vi "MGI Dispose Daemon.vi"(11 "MGI Error Reporter Base In":refnum<class "MGI Error Reporter Base.lvclass">) -> (3 "MGI Error Reporter Base Out":refnum<class "MGI Error Reporter Base.lvclass">)   [LabVIEW 2020, in "MGI Error Reporter Base.lvclass"]
doc: "Releases the specified references. Child classes can perform other tasks as appropriate, but should use Call Parent Method before completing.\n\nAuthored by Shawn Walpole\nsupport@mooregoodideas.com\nwww.mooregoodideas.com\n\nCopyright (c) 2013, Moore Good Ideas, Inc.\n\nAll rights reserved.\n\nRedistribution and use in source and binary forms, with or without modification, are permitted provided that the following conditions are met:\n\n * Redistributions of source code must retain the above copyright notice, this list of conditions and the following disclaimer.\n * Redistributions in binary form must reproduce the above copyright notice, this list of conditions and the following disclaimer in the documentation and/or other materials provided with the distribution.\n * Neither the name of Moore Good Ideas, Inc. nor the names of its contributors may be used to endorse or promote products derived from this software without specific prior written permission.\n\nTHIS SOFTWARE IS PROVIDED BY THE COPYRIGHT HOLDERS AND CONTRIBUTORS \"AS IS\" AND ANY EXPRESS OR IMPLIED WARRANTIES, INCLUDING, BUT NOT LIMITED TO, THE IMPLIED WARRANTIES OF MERCHANTABILITY AND FITNESS FOR A PARTICULAR PURPOSE ARE DISCLAIMED. IN NO EVENT SHALL THE COPYRIGHT OWNER OR CONTRIBUTORS BE LIABLE FOR ANY DIRECT, INDIRECT, INCIDENTAL, SPECIAL, EXEMPLARY, OR CONSEQUENTIAL DAMAGES (INCLUDING, BUT NOT LIMITED TO, PROCUREMENT OF SUBSTITUTE GOODS OR SERVICES; LOSS OF USE, DATA, OR PROFITS; OR BUSINESS INTERRUPTION) HOWEVER CAUSED AND ON ANY THEORY OF LIABILITY, WHETHER IN CONTRACT, STRICT LIABILITY, OR TORT (INCLUDING NEGLIGENCE OR OTHERWISE) ARISING IN ANY WAY OUT OF THE USE OF THIS SOFTWARE, EVEN IF ADVISED OF THE POSSIBILITY OF SUCH DAMAGE."
uses:
  <userlib>/_MGI/Error Reporter/MGI Error Reporter Base/MGI Error Reporter Base.lvclass
  <userlib>/_MGI/Error Reporter/MGI Error Reporter Base/MGI Error Reporter Base.lvclass/MGI Error Reporter Base.ctl
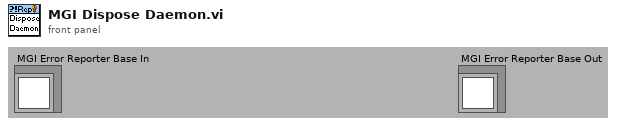
[diagram p1: front panel]
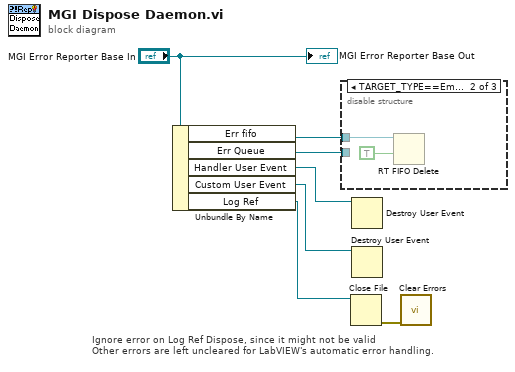
[diagram p0: block diagram]
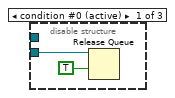
[diagram p2: hidden frame]
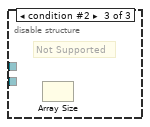
[diagram p3: hidden frame]
diagram:
  # "Ignore error on Log Ref Dispose, since it might not be valid\nOther errors are left uncleared for LabVIEW's automatic error handling."
  n1 = Unbundle By Name("MGI Error Reporter Base In") -> ("Err fifo"=w1:refnum<k33>, "Err Queue"=w6:refnum<queue>, "Handler User Event"=w5:refnum<user-event>, "Custom User Event"=w4:refnum<user-event>, "Log Ref"=w2:refnum<file>)
  n2 = disable-structure shown="TARGET_TYPE==Embedded||TARGET_TYPE==RT" {
    disable-tunnel: w6 -> [w8 _ _]
    disable-tunnel: w1 -> [_ w11 _]
    frame condition #0 (active) {
      n3 = Release Queue(queue=w8, force destroy? (F)=TRUE) -> ()  [unwired: 1 in, 3 out]
    }
    frame condition #1 {
      n4 = RT FIFO Delete(0:w11, 2:TRUE ("force destroy? (F)")) -> ()  [unwired: 1 in, 1 out]
    }
    frame condition #2 {
      # "Not Supported"
      n5 = Array Size() -> ()  [unwired: 1 in, 1 out]
    }
  }
  n6 = Close File(refnum=w2) -> (error out=w3:errorcluster)  [unwired: 1 in, 1 out]
  n7 = Destroy User Event(user event=w5) -> ()  [unwired: 1 in, 1 out]
  n8 = Destroy User Event(user event=w4) -> ()  [unwired: 1 in, 1 out]
  n9 = call <vilib>:"Clear Errors.vi"("error in (no error)"=w3) -> ()  [unwired: 1 in, 6 out]
  "MGI Error Reporter Base Out" <- "MGI Error Reporter Base In"
